vi "USB grab (SubVI).vi"(8 "error in (no error)":errorcluster, 10 "logfile base name in":string="logfile", 11 "Numeric":i32) -> (0 "error out":errorcluster, 3 "Refnum out":T1(plugin-control))   [LabVIEW 2018]
uses:
  <vilib>/vision/driver/Vision Acquisition Express Utility VIs.llb/Vision Acquisition Path Convert (Path).vi
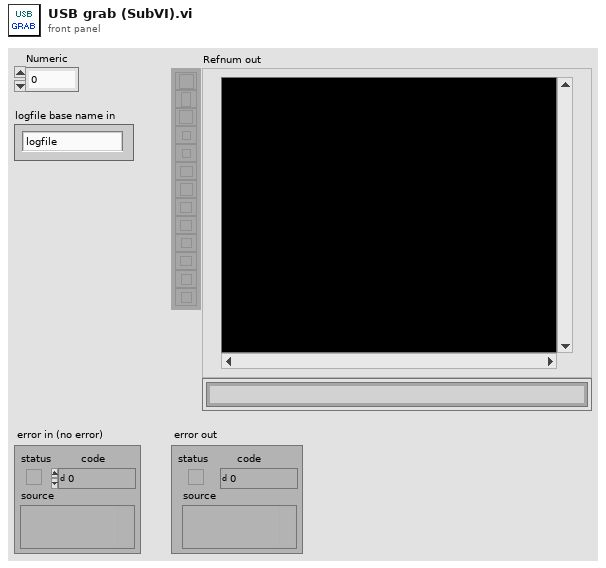
[diagram p1: front panel]
types:
  T1 = typedef "IMAQ Image.ctl" = refnum<image>
  T2 = typedef "Image Type" = u32
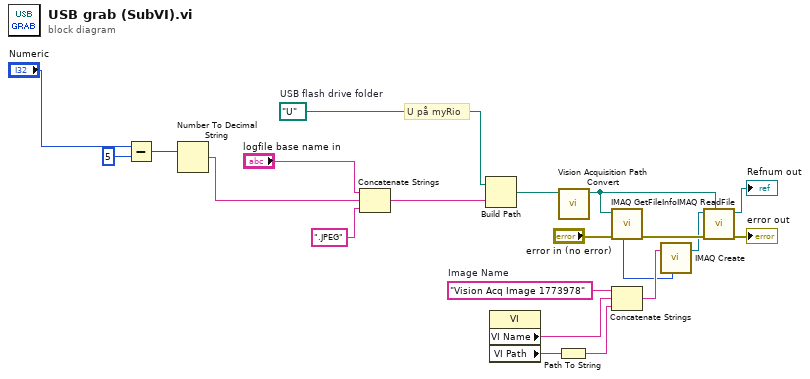
[diagram p0: block diagram]
diagram:
  w16 = "Vision Acq Image 1773978"  # Image Name
  w4 = path "U:/"  # USB flash drive folder
  # "U på myRio"
  n1 = Subtract(x="Numeric", y=5) -> (x-y=w1:i32)
  n2 = Number To Decimal String(number=w1) -> (decimal integer string=w21:string)  [unwired: 1 in]
  n3 = Concatenate Strings "Concatenate Strings"("logfile base name in", w21, ".JPEG" ("string")) -> (w6:string)
  n4 = Build Path(base path=w4, name or relative path=w6) -> (appended path=w20:path)
  n5 = property class="VI"() -> ("VI Name"=w14:string, "VI Path"=w13:path)  [unwired: 2 in, 2 out]
  n6 = Path To String(path=w13) -> (string=w15:string)
  n7 = call-poly <vilib>:"Vision Acquisition Path Convert.vi"("Path In"=w20) -> ("Path Out"=w19:path)  [unwired: 10 in]
  n8 = call "IMAQ GetFileInfo"("error in (no error)"="error in (no error)", "File Path"=w19) -> ("error out"=w12:errorcluster, "Image Type"=w10:T2)  [unwired: 8 out]
  n9 = Concatenate Strings(w16, w14, w15) -> (w17:string)
  n10 = call "IMAQ Create"("Image Name"=w17, "Image Type"=w10) -> ("New Image"=w8:T1)  [unwired: 2 in, 2 out]
  n11 = call "IMAQ ReadFile"("File Path"=w19, "error in (no error)"=w12, "Image"=w8) -> ("error out"=→"error out":errorcluster, "Image Out"=→"Refnum out":T1)  [unwired: 2 in, 5 out]
